vi "filterWfmsButterworthBandpass.vi"(0 "Instrument handle":refnum<k15>, 1 "Reset filters":bool, 5 "Q factor":i32=2, 7 "F0":dbl format="%.2p", 9 "Order":i32=2, 11 "error in (no error)":errorcluster, 12 "Time signal(s) in":waveform(dbl)[](array[waveform])) -> (4 "Instrument handle out":refnum<k15>, 6 "Filter information":T1, 14 "Filtered time signal(s)":waveform(dbl)[](array[waveform]), 15 "error out":errorcluster)   [LabVIEW 2020]
uses:
  <vilib>/measure/macond.llb/IIR Filter for N Chan.vi
  <vilib>/measure/NI_MAPro.lvlib
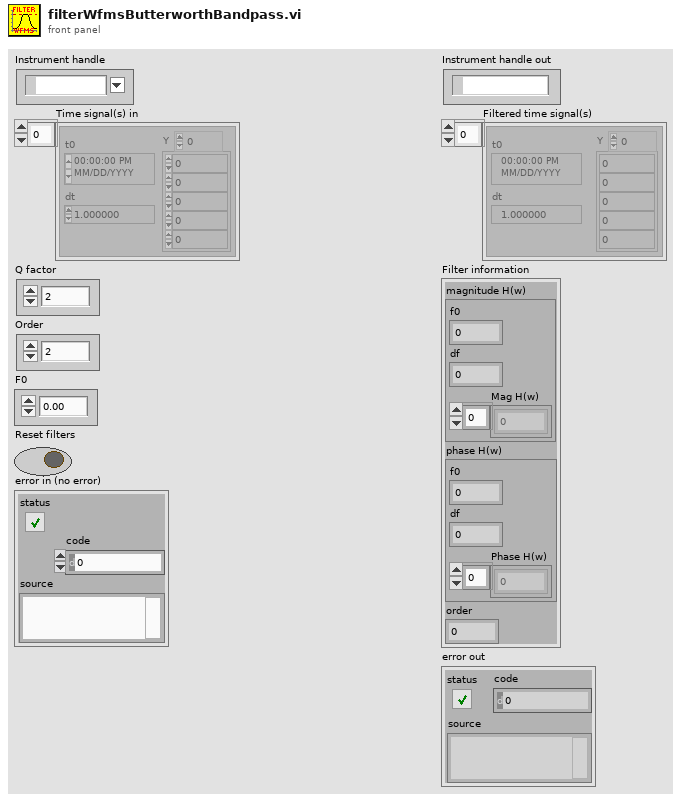
[diagram p1: front panel]
types:
  T1 = cluster{"magnitude H(w)":cluster{"f0":dbl, "df":dbl, "Mag H(w)":dbl[]}, "phase H(w)":cluster{"f0":dbl, "df":dbl, "Phase H(w)":dbl[]}, "order":i32}
  T2 = enum16{"Off", "Butterworth", "Chebyshev", "Inverse Chebyshev", "Elliptic", "Bessel"}
  T3 = enum16{"Lowpass", "Highpass", "Bandpass", "Bandstop"}
  T4 = cluster{"Topology":enum16{"Off", "Butterworth", "Chebyshev", "Inverse Chebyshev", "Elliptic", "Bessel"}, "Type":enum16{"Lowpass", "Highpass", "Bandpass", "Bandstop"}, "Order":i32, "Lower Fc":dbl, "Upper Fc":dbl, "PB Ripple":dbl, "SB Attenuation":dbl}
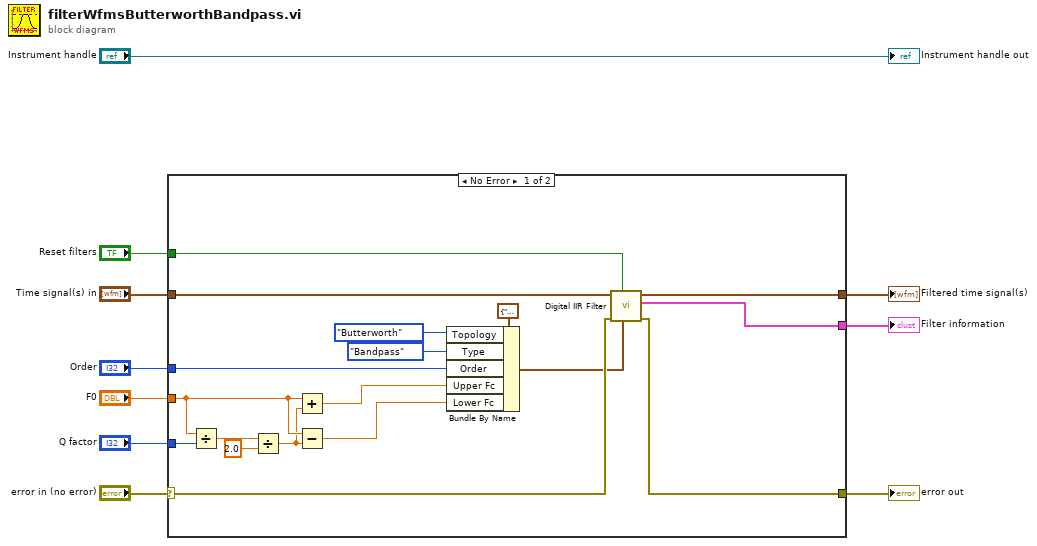
[diagram p0: block diagram]
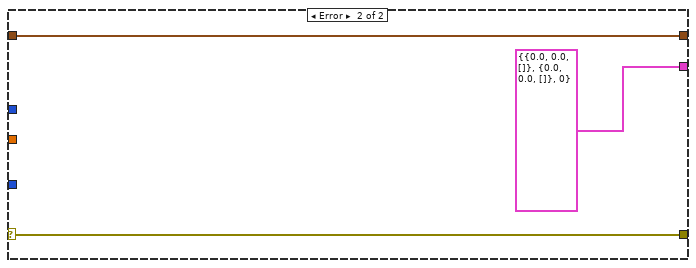
[diagram p2: hidden frame]
diagram:
  n1 = case shown="No Error" "error in (no error)" {
    selector: "error in (no error)" -> [w22 w31]
    tunnel: "Time signal(s) in" -> [w23 w29]
    tunnel: "Order" -> [w16 _]
    tunnel: "Q factor" -> [w28 _]
    tunnel: "F0" -> [w27 _]
    tunnel: [w21 w31] -> w4
    tunnel: [w20 w29] -> w5
    tunnel: "Reset filters" -> [w12 _]
    tunnel: [w11 T1 {"magnitude H(w)"={"f0"=0.0, "df"=0.0, "Mag H(w)"=[]}, "phase H(w)"={"f0"=0.0, "df"=0.0, "Phase H(w)"=[]}, "order"=0} ("filter information")] -> w1
    frame No Error {
      n2 = Divide(x=w27, y=w28) -> (x/y=w26:dbl)
      n3 = Divide(x=w26, y=2.0) -> (x/y=w25:dbl)
      n4 = Add(x=w27, y=w25) -> (x+y=w15:dbl)
      n5 = Subtract(x=w27, y=w25) -> (x-y=w14:dbl)
      n6 = Bundle By Name(cluster=T4 {"Topology"=enum."Butterworth", "Type"=enum."Lowpass", "Order"=1, "Lower Fc"=100.0, "Upper Fc"=200.0, "PB Ripple"=1.0, "SB Attenuation"=60.0} ("IIR filter specifications"), "Topology"=T2."Butterworth", "Type"=T3."Bandpass", "Order"=w16, "Upper Fc"=w15, "Lower Fc"=w14) -> (w13:T4)
      n7 = call-poly <vilib>:"Digital IIR Filter.vi"("IIR filter specifications"=w13, "reset filters"=w12, "error in (no error)"=w22, "signal(s) in"=w23) -> ("error out"=w21:errorcluster, "filter information"=w11:T1, "signal(s) out"=w20:waveform(dbl)[])  [unwired: 5 in]
    }
    frame Error {
    }
  }
  "Filtered time signal(s)" <- w5
  "error out" <- w4
  "Filter information" <- w1
  "Instrument handle out" <- "Instrument handle"
